vi "Packets and Groups.vi"(8 "Iteration Treshold Time [sec]":dbl, 9 "Packet Size":i16, 10 "Duration [sec]":dbl=1.0, 11 "Acquisition Rate":i16(ring)=10 items=["10"=10, "15"=15, "20"=20, "25"=25, "30"=30, "40"=40, "45"=45, "50"=50, "60"=60, "75"=75, "80"=80, "90"=90, "100"=100, "120"=120, "125"=125, "150"=150, "180"=180, "200"=200, "225"=225, "240"=240, "250"=250, "300"=300, "360"=360, "400"=400, "450"=450, "500"=500, "600"=600, "800"=800, "900"=900, "1000"=1000, "1200"=1200, "1500"=1500, "1800"=1800, "2000"=2000]) -> (0 "ACTUAL DURATION":dbl=1.6, 1 "Iteration Time [sec]":dbl=1.6, 2 "GROUPS":i32=1, 3 "PACKETS":i32=1)   [LabVIEW 2015, in "G 5.lvlib"]
uses:
  G 5.lvlib
panel:
  out "Packets Calc":dbl
  out "GROUPS Calc":dbl=0.625
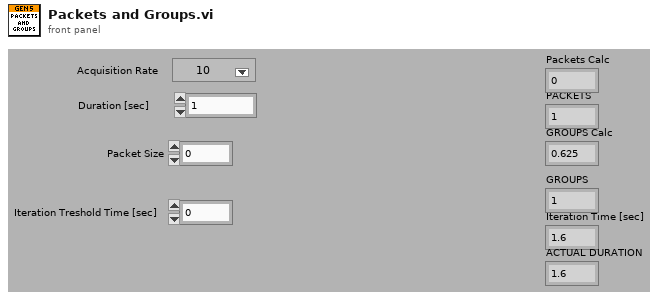
[diagram p1: front panel]
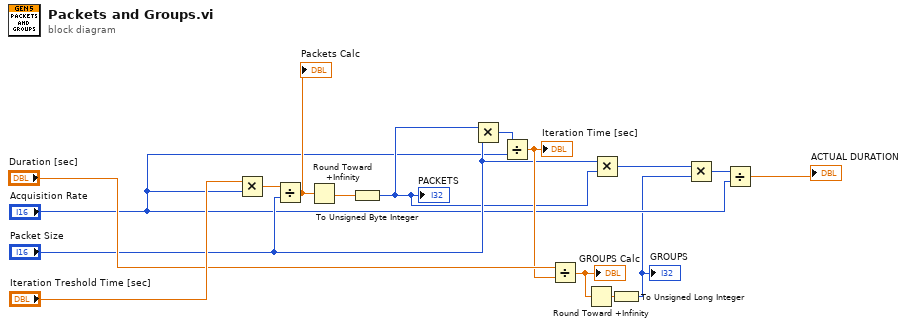
[diagram p0: block diagram]
diagram:
  n1 = Multiply(x="Iteration Treshold Time [sec]", y="Acquisition Rate") -> (x*y=w15:dbl)
  n2 = Divide(x=w15, y="Packet Size") -> (x/y=w13:dbl)
  "Packets Calc" <- w13
  n3 = Round Toward +Infinity(x=w13) -> (ceil(x): smallest int >= x=w14:dbl)
  n4 = To Unsigned Byte Integer(number=w14) -> (unsigned 8bit integer=w6:u8)
  "PACKETS" <- w6
  n5 = Multiply(x=w6, y="Packet Size") -> (x*y=w12:i16)
  n6 = Divide(x=w12, y="Acquisition Rate") -> (x/y=w10:dbl)
  "Iteration Time [sec]" <- w10
  n7 = Divide(x="Duration [sec]", y=w10) -> (x/y=w9:dbl)
  "GROUPS Calc" <- w9
  n8 = Round Toward +Infinity(x=w9) -> (ceil(x): smallest int >= x=w8:dbl)
  n9 = Multiply(x="Packet Size", y=w6) -> (x*y=w4:i16)
  n10 = To Unsigned Long Integer(number=w8) -> (unsigned 32bit integer=w3:u32)
  "GROUPS" <- w3
  n11 = Multiply(x=w4, y=w3) -> (x*y=w2:u32)
  n12 = Divide(x=w2, y="Acquisition Rate") -> (x/y=→"ACTUAL DURATION":dbl)
